vi "Get Parent.vi"(11 "Path":string) -> (3 "parent":string)   [LabVIEW 2018]
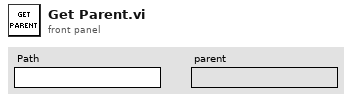
[diagram p1: front panel]
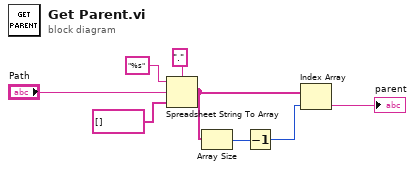
[diagram p0: block diagram]
diagram:
  n1 = Spreadsheet String To Array(delimiter (Tab)=".", format string="%s", spreadsheet string="Path", array type (2D Dbl)=string[] []) -> (array=w3:string[])
  n2 = Array Size(array=w3) -> (size(s)=w4:i32)
  n3 = Decrement(x=w4) -> (x-1=w5:i32)
  n4 = Index Array(array=w3, index=w5) -> (element=→"parent":string)
